vi "while_v0_v22.vi"() -> ()   [LabVIEW 2010]
panel:
  in  "Width 1":dbl(knob)=20.0 scale=0.0..20.0
  in  "Width 0":dbl(knob)=5.636149259871094 scale=0.0..20.0
  out "Waveform Chart":dbl(graph)
  in  "Delay (ms)":dbl(slide)=25.71428571428571 scale=0.0..300.0
  out "Secventa":i64=5
  in  "stop":bool
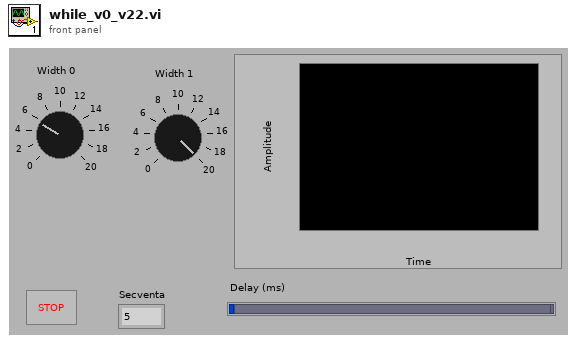
[diagram p1: front panel]
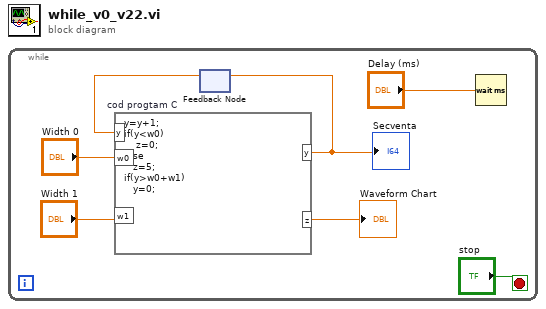
[diagram p0: block diagram]
diagram:
  n1 = while {
    stop <- "stop" stop-if-true
    n2 = feedback #1() -> (w1:dbl)  [unwired: 1 in]
    n3 = formula code="y=y+1;\nif(y<w0)\n    z=0;\nelse\n   z=5;\nif(y>w0+w1)\n   y=0;" "cod progtam C"("w0"="Width 0", "w1"="Width 1", "y"=w1) -> ("y"=w2:dbl, "z"=→"Waveform Chart":dbl)
    "Secventa" <- w2
    n4 = feedback-in #1(w2) -> ()
    n5 = Wait (ms)(milliseconds to wait="Delay (ms)") -> ()  [unwired: 1 out]
  }
